vi "carrier_waveforms.vi"(5 "Modulation info":T8={"Fs full"=0.0, "Fs high"=0.0, "Fs low"=0.0, "Read size"=0, "FFT size low"=5000, "df low"=5000.0, "High carriers"=[], "Low carriers"=[], "Hi channels at low"=[7]} {"Hi channels at low" min=0 step=1; "Low carriers" format="%#_6p"; "High carriers" format="%#_6p"}, 6 "Freq response":bool, 7 "ilemt_config":T2={"IO params"={"Conversion"={"Rate"=4.0, "Num cards"=2, "Out channels"=4}, "Carriers"={"Phase shift"=180.0, "Levels"=[[0.8, 0.8, 0.8], [0.03, 0.03, 0.03]], "Delay samples"=73.15}, "TCP"={"Host"="192.168.1.15", "Port"=6666, "Buffering"=6, "Timeout"=6}, "Input channel sign"=[1, 1, 1]}, "High rate STFT"={"Win param"=101.5, "Window type"=61, "Win order"=2, "DFT size"=64, "Channels"=[7], "Oversample"=64}, "Low rate STFT"={"Win param"=120.0, "Window type"=61, "Win order"=8, "DFT size"=64, "Channels"=[7], "Oversample"=64}, "Filtering "=[]} {"Filtering"."Distortion"."Limit" format="%#_3p"; "Filtering"."Distortion"."LF cut" format="%#_3p"; "Filtering"."Kalman"."Measure noise" format="%#_3p"; "Filtering"."Kalman"."Process noise" format="%#_3p"; "Filtering"."Hum"."Limit" format="%#_3p"; "Filtering"."Hum"."Frequency" format="%#_4p"; "Low rate STFT"."Oversample" min=1 step=1; "Low rate STFT"."Channels" min=0 step=1; "Low rate STFT"."DFT size" min=1 step=1; "Low rate STFT"."Window type" items=["Rectangle"=0, "Hanning"=1, "Hamming"=2, "Blackman-Harris"=3, "Exact Blackman"=4, "Blackman"=5, "Flat Top"=6, "4 Term B-Harris "=7, "7 Term B-Harris"=8, "Low Sidelobe"=9, "Blackman Nuttall"=11, "Triangle"=30, "Bartlett-Hanning"=31, "Bohman"=32, "Parzen"=33, "Welch"=34, "Kaiser"=60, "Dolph-Chebyshev"=61, "Gaussian"=62]; "High rate STFT"."Oversample" min=1 step=1; "High rate STFT"."Channels" min=0 step=1; "High rate STFT"."DFT size" min=1 step=1; "High rate STFT"."Window type" items=["Rectangle"=0, "Hanning"=1, "Hamming"=2, "Blackman-Harris"=3, "Exact Blackman"=4, "Blackman"=5, "Flat Top"=6, "4 Term B-Harris "=7, "7 Term B-Harris"=8, "Low Sidelobe"=9, "Blackman Nuttall"=11, "Triangle"=30, "Bartlett-Hanning"=31, "Bohman"=32, "Parzen"=33, "Welch"=34, "Kaiser"=60, "Dolph-Chebyshev"=61, "Gaussian"=62]; "IO params"."Input channel sign" min=-1 max=1 step=1; "IO params"."Carriers"."Levels" min=0.0 step=0.1; "IO params"."Conversion"."Rate" format="%#_8g"}) -> (1 "Comp fault":bool, 2 "Output data":i32[][](array[numeric]), 3 "Source waveforms":waveform(dbl)[](graph))   [LabVIEW 2024]
uses:
  modulation_info.ctl
  ilemt_config.ctl
  system/IO_params.ctl
  stft_params.ctl
  <vilib>/Analysis/4window.llb/windowTd.ctl
  filter_params.ctl
  detrend_mode.ctl
  card_carrier_amplitudes.ctl
  <vilib>/Analysis/2dsp.llb/Inverse Real FFT.vi
  main/ilemt_globals.vi
  <vilib>/measure/NI_MABase.lvlib
  <vilib>/Analysis/NI_AALPro.lvlib
panel:
  in  "Comp fault threshold":dbl=0.2
  in  "Comp gain":dbl=0.05
  in  "Comp once":bool
  out "Compensated output":T1=[[[0.8395770614877774+0.0028758063900550953i, -0.018324423372348016-0.0006201934581264143i, -0.016886925649108726-2.940545835293518e-05i], [-0.01697562432214083-0.0016348024111330225i, 0.83885135156083+0.0020670504279334634i, -0.017173180533270275+0.00019269400281305392i], [-0.016374422884271427-0.0030083353945267676i, -0.0193629198646361-0.0014643391916366435i, 0.8367125904896281-0.0010501471602728106i]], [[0.03133897239102365+0.0006252328873188348i, -0.00048275091331450914-0.0003089130018055452i, -0.00043021631765542174-0.0002759884878732777i], [-0.0005913630072077795-0.00031200916130722737i, 0.03127992971510062+0.0004833529231568414i, -0.000494785304455945-0.0002579575827334465i], [-0.0007333860538198184-0.0003567516731933187i, -0.0006880917601750341-0.00033092556285938983i, 0.031083261126587918+0.00032228091837395326i]]] format="%#_3p"
  in  "Coupling comp":bool=TRUE
  # "Frequency response calibration mode"
  # "Parameters:"
  # "Gain used by auto-compensation of carrier cross coupling, <= 1. This is an integral gain."
  # "What fraction of the total carrier amplitude that the compensated carrier amplitude may differ from the uncompensated carrier amplitudes."
  # "Compensation on?"
  # "Trigger a compensation now, at gain 1."
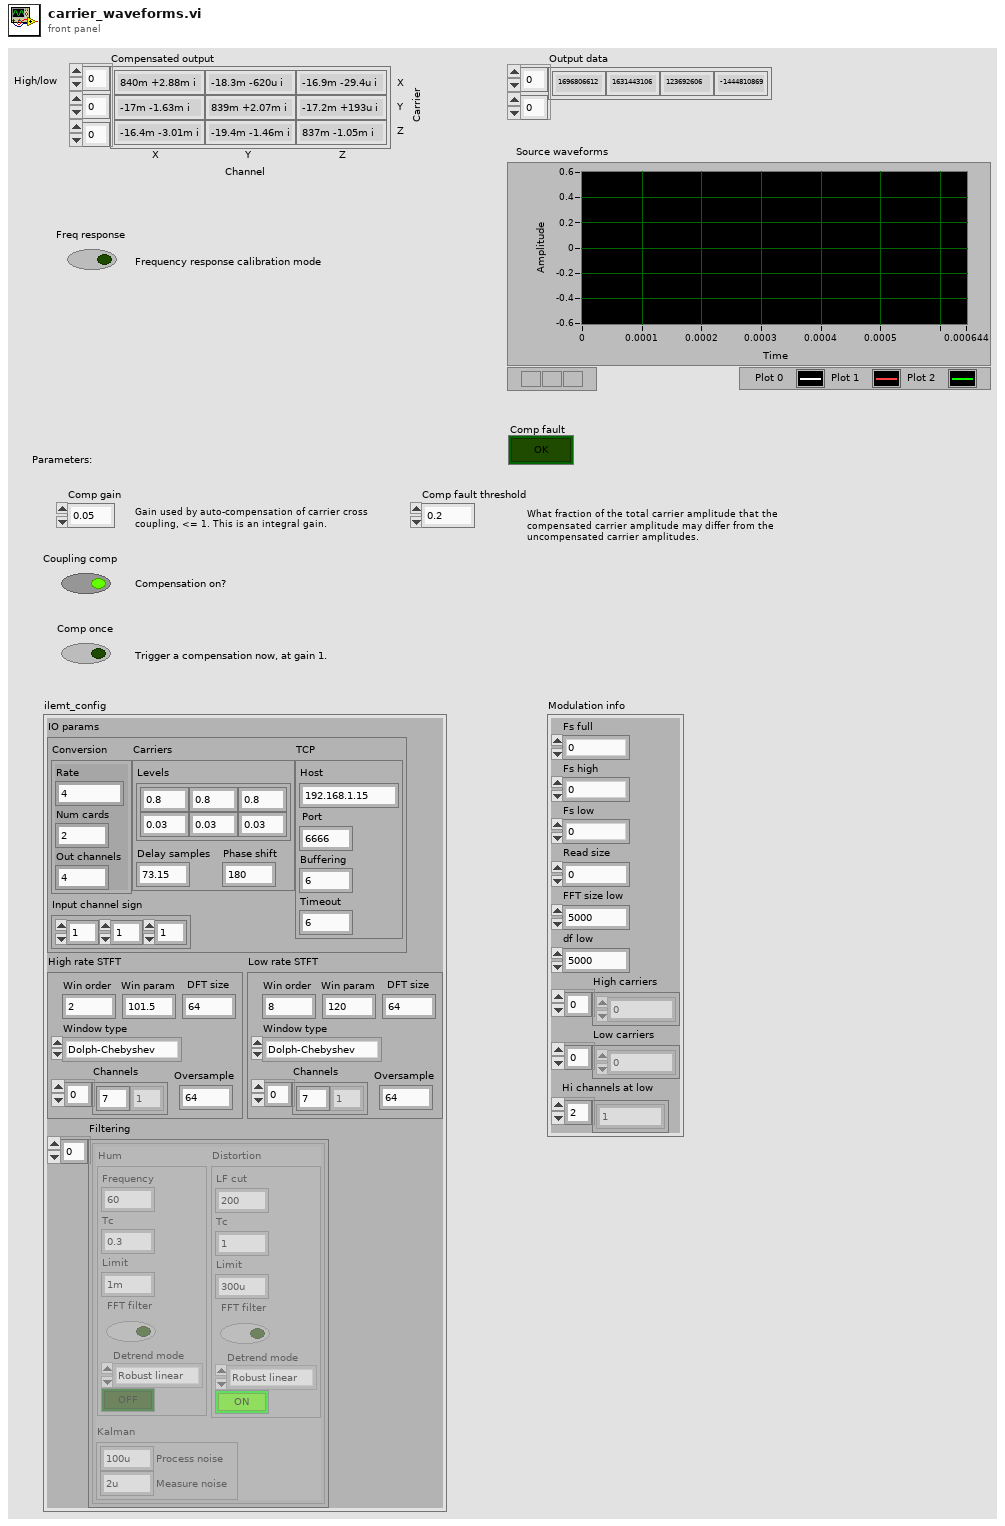
[diagram p1: front panel]
types:
  T1 = typedef "card_carrier_amplitudes.ctl" = cdb[][][]
  T2 = typedef "ilemt_config.ctl" = cluster{"IO params":T3, "High rate STFT":T4, "Low rate STFT":T4, "Filtering ":T6[]}
  T3 = typedef "IO_params.ctl" = cluster{"Conversion":cluster{"Rate":dbl, "Num cards":u32, "Out channels":u32}, "Carriers":cluster{"Phase shift":dbl, "Levels":dbl[][], "Delay samples":dbl}, "TCP":cluster{"Host":string, "Port":i32, "Buffering":u32, "Timeout":u32}, "Input channel sign":i32[]}
  T4 = typedef "stft_params.ctl" = cluster{"Win param":dbl, "Window type":T5, "Win order":i32, "DFT size":i32, "Channels":i32[], "Oversample":i32}
  T5 = typedef "NI_AALPro.lvlib/windowTd.ctl" = u32
  T6 = typedef "filter_params.ctl" = cluster{"Hum":cluster{"Frequency":dbl, "Tc":dbl, "Limit":dbl, "FFT filter":bool, "Detrend mode":T7, "Enable":bool}, "Kalman":cluster{"Process noise":dbl, "Measure noise":dbl}, "Distortion":cluster{"LF cut":dbl, "Tc":dbl, "Limit":dbl, "FFT filter":bool, "Detrend mode":T7, "Enable":bool}}
  T7 = typedef "detrend_mode.ctl" = enum16{"Zero mean", "Linear", "Robust linear"}
  T8 = typedef "modulation_info.ctl" = cluster{"Fs full":dbl, "Fs high":dbl, "Fs low":dbl, "Read size":i32, "FFT size low":i32, "df low":dbl, "High carriers":dbl[], "Low carriers":dbl[], "Hi channels at low":i32[]}
  T9 = typedef "carrier_amplitudes.ctl" = cdb[][][][]
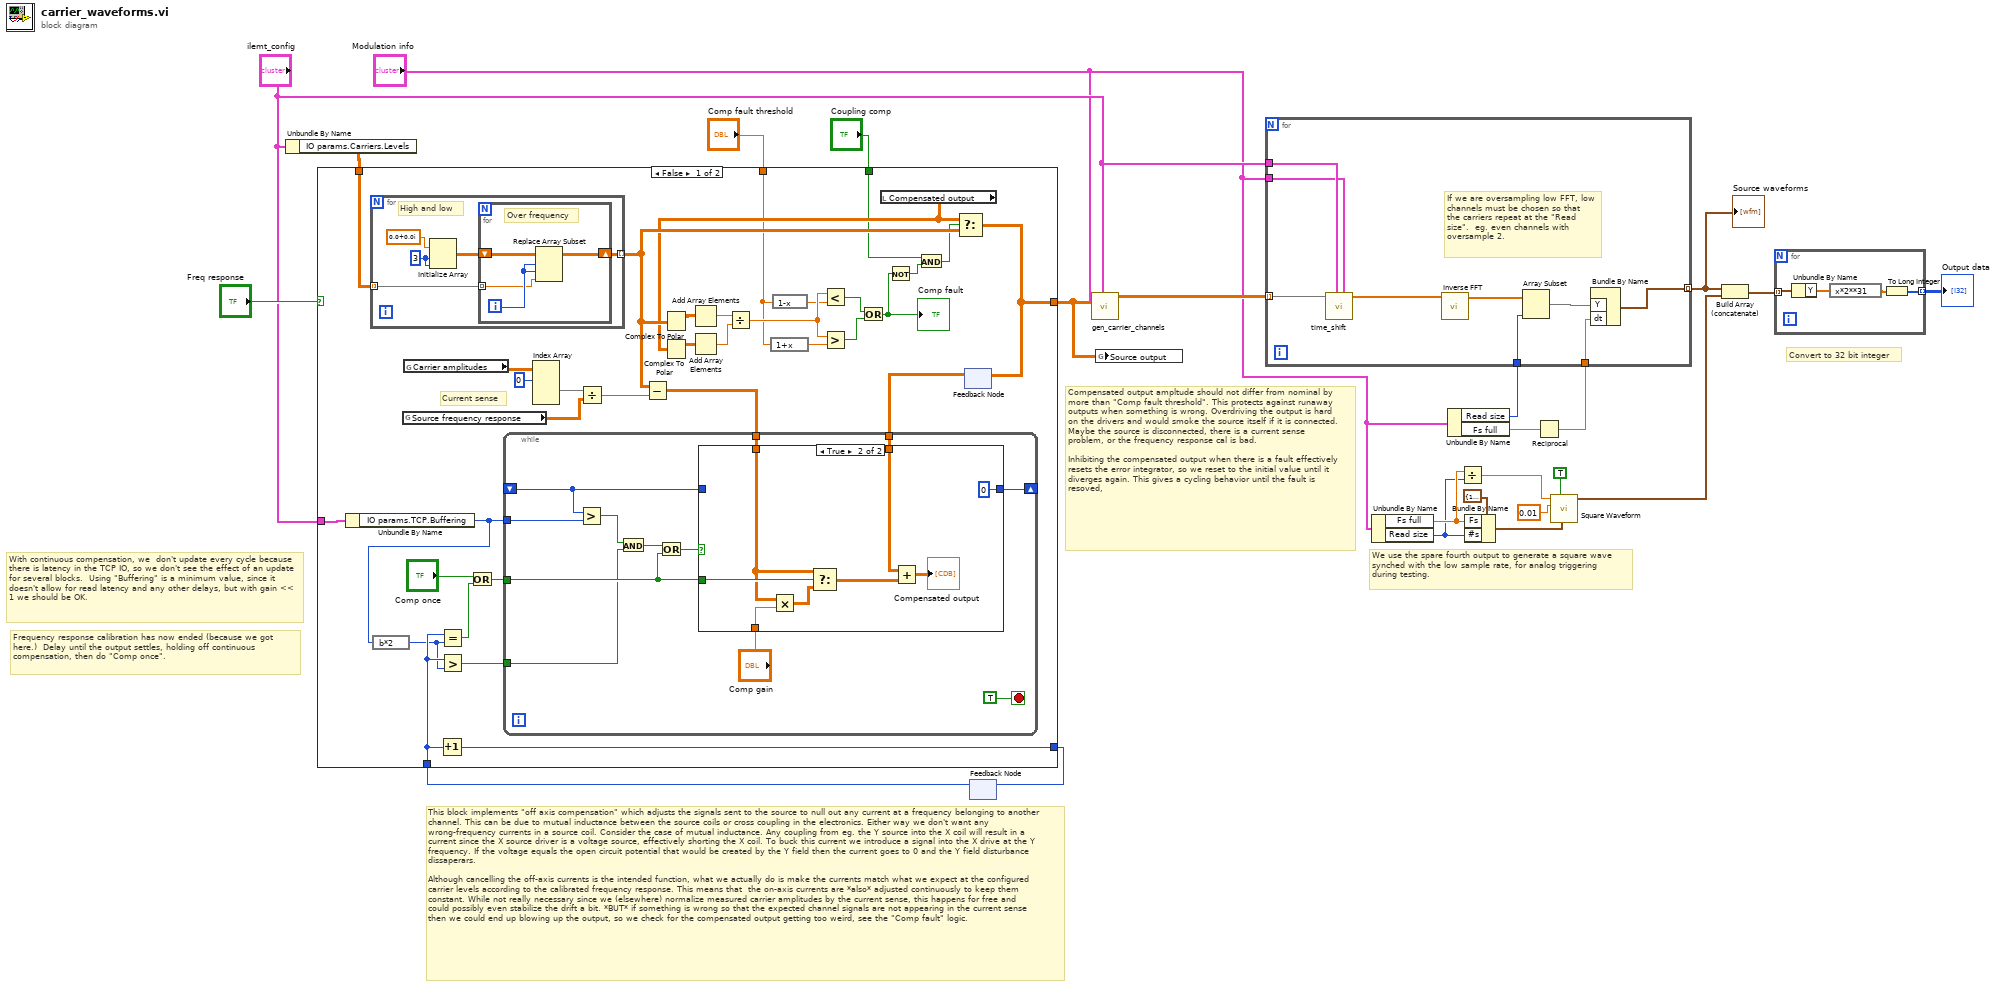
[diagram p0: block diagram]
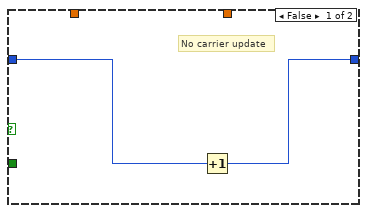
[diagram p2: hidden frame]
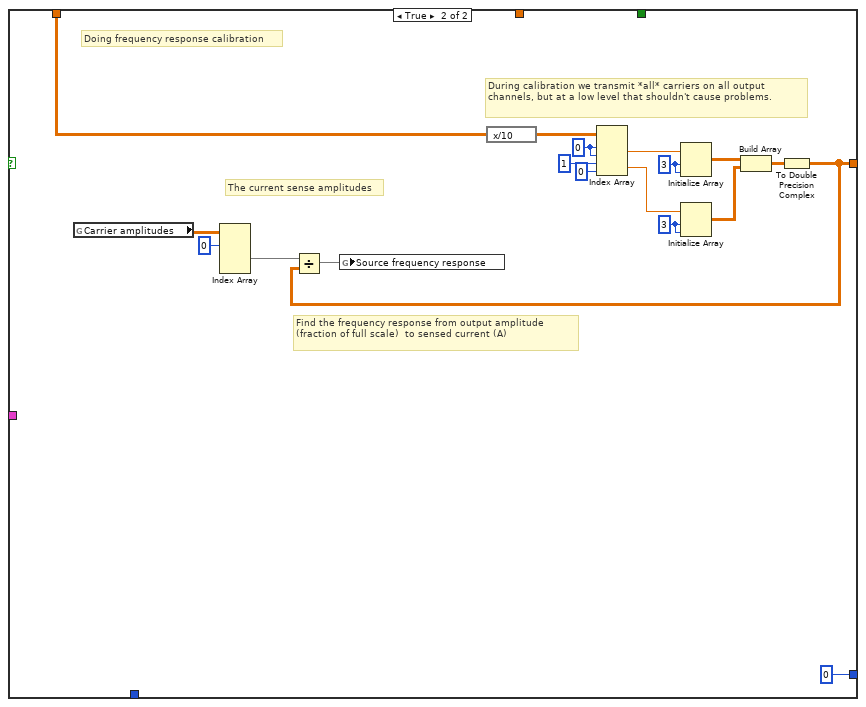
[diagram p3: hidden frame]
diagram:
  # "This block implements \"off axis compensation\" which adjusts the signals sent to the source to null out any current at a frequency belonging to another channel. This can be due to mutual inductance between the source coils or cross coupling in the electronics. Either way we don't want any wrong-frequency currents in a source coil. Consider the case of mutual inductance. Any coupling from eg. the Y source into the X coil will result in a current since the X source driver is a voltage source, effectively shorting the X coil. To buck this current we introduce a signal into the X drive at the Y frequency. If the voltage equals the open circuit potential that would be created by the Y field then the current goes to 0 and the Y field disturbance dissaperars.\n\nAlthough cancelling the off-axis currents is the intended function, what we actually do is make the currents match what we expect at the configured carrier levels according to the calibrated frequency response. This means that  the on-axis currents are *also* adjusted continuously to keep them constant. While not really necessary since we (elsewhere) normalize measured carrier amplitudes by the current sense, this happens for free and could possibly even stabilize the drift a bit. *BUT* if something is wrong so that the expected channel signals are not appearing in the current sense then we could end up blowing up the output, so we check for the compensated output getting too weird, see the \"Comp fault\" logic."
  # "Compensated output ampltude should not differ from nominal by more than \"Comp fault threshold\". This protects against runaway outputs when something is wrong. Overdriving the output is hard on the drivers and would smoke the source itself if it is connected. Maybe the source is disconnected, there is a current sense problem, or the frequency response cal is bad.\n\nInhibiting the compensated output when there is a fault effectively resets the error integrator, so we reset to the initial value until it diverges again. This gives a cycling behavior until the fault is resoved,"
  # "Frequency response calibration has now ended (because we got here.)  Delay until the output settles, holding off continuous compensation, then do \"Comp once\"."
  # "With continuous compensation, we  don't update every cycle because there is latency in the TCP IO, so we don't see the effect of an update for several blocks.  Using \"Buffering\" is a minimum value, since it doesn't allow for read latency and any other delays, but with gain << 1 we should be OK."
  # "Convert to 32 bit integer"
  # "We use the spare fourth output to generate a square wave synched with the low sample rate, for analog triggering during testing."
  n1 = Unbundle By Name("ilemt_config") -> ("IO params.Carriers.Levels"=w9:dbl[][])
  n2 = feedback #1() -> (w4:i32)  [unwired: 1 in]
  n3 = case shown="False" "Freq response" {
    tunnel: w9 -> [w58 w92]
    tunnel: [w53 w90] -> w7
    tunnel: "ilemt_config" -> [w52 _]
    tunnel: [w50 0 ("Read size")] -> w5
    tunnel: w4 -> [w45 _]
    tunnel: "Coupling comp" -> [w28 _]
    tunnel: "Comp fault threshold" -> [w25 _]
    frame False {
      # "Current sense"
      n4 = Unbundle By Name(w52) -> ("IO params.TCP.Buffering"=w49:u32)
      n5 = for {
        tunnel: w58 -> [w82] mode=indexing
        tunnel: [w81] -> w40 mode=indexing
        w85 = 3 ("dimension size")
        # "High and low"
        n6 = Initialize Array(cdb 0.0+0.0i, w85, w85) -> (w83:cdb[][])
        n7 = for {
          tunnel: w82 -> [w87] mode=indexing
          shift-right: [w86] -> w81
          shift-left: w83 -> [w89]
          i -> [w88]
          # "Over frequency"
          n8 = Replace Array Subset(array=w89, new element=w87, index (row)=w88, index (col)=w88) -> (w86:cdb[][])
        }
      }
      n9 = expression code="b*2"(w49) -> (w44:u32)
      n10 = global read "ilemt_globals.vi" "Source frequency response"() -> (w54:T1)
      n11 = global read "ilemt_globals.vi" "Carrier amplitudes"() -> (w57:T9)
      n12 = Increment(x=w45) -> (x+1=w50:i32)
      n13 = Equal?(x=w45, y=w44) -> (x = y?=w47:bool)
      n14 = Greater?(x=w45, y=w44) -> (0:w43:bool)
      n15 = Or(x="Comp once", y=w47) -> (x .or. y?=w46:bool)
      n16 = Index Array(array=w57, index (dim 0)=0 ("index (vol)")) -> (element=w55:cdb[][][])  [unwired: 3 in]
      n17 = Divide(x=w55, y=w54) -> (x/y=w37:cdb[][][])
      n18 = Subtract(x=w40, y=w37) -> (x-y=w51:cdb[][][])
      n19 = Complex To Polar(r * e^(i*theta)=w40) -> (r=w39:dbl[][][])  [unwired: 1 out]
      n20 = Add Array Elements(numeric array=w39) -> (sum=w42:dbl)
      n21 = expression code="1+x"(w25) -> (w27:dbl)
      n22 = expression code="1-x"(w25) -> (w26:dbl)
      n23 = local read "Compensated output"() -> (w29:T1)
      n24 = Complex To Polar(r * e^(i*theta)=w29) -> (r=w38:dbl[][][])  [unwired: 1 out]
      n25 = Add Array Elements(numeric array=w38) -> (sum=w41:dbl)
      n26 = Divide(x=w42, y=w41) -> (x/y=w36:dbl)
      n27 = Less?(x=w36, y=w26) -> (x < y?=w34:bool)
      n28 = Greater?(x=w36, y=w27) -> (0:w35:bool)
      n29 = Or(x=w34, y=w35) -> (x .or. y?=w33:bool)
      "Comp fault" <- w33
      n30 = Not(x=w33) -> (.not. x?=w32:bool)
      n31 = And(x=w28, y=w32) -> (x .and. y?=w31:bool)
      n32 = Select(t=w29, s=w31, f=w40) -> (s? t:f=w53:T1)
      n33 = feedback-in #2(w53) -> ()
      n34 = feedback #2() -> (w30:T1)  [unwired: 1 in]
      n35 = while {
        tunnel: w46 -> [w65]
        shift-right: [w67] -> _
        shift-left: _ -> [w68]
        tunnel: w49 -> [w69]
        tunnel: w30 -> [w66]
        tunnel: w51 -> [w64]
        tunnel: w43 -> [w60]
        stop <- TRUE stop-if-true
        n36 = Greater?(x=w68, y=w69) -> (0:w62:bool)
        n37 = And(x=w62, y=w60) -> (x .and. y?=w61:bool)
        n38 = Or(x=w61, y=w65) -> (x .or. y?=w59:bool)
        n39 = case shown="True" w59 {
          tunnel: w68 -> [w72 _]
          tunnel: [w71 0] -> w67
          tunnel: w66 -> [_ w79]
          tunnel: w65 -> [_ w77]
          tunnel: w64 -> [_ w75]
          tunnel: "Comp gain" -> [_ w73]
          frame False {
            # "No carrier update"
            n40 = Increment(x=w72) -> (x+1=w71:i32)
          }
          frame True {
            n41 = Multiply(x=w75, y=w73) -> (x*y=w74:cdb[][][])
            n42 = Select(t=w75, s=w77, f=w74) -> (s? t:f=w76:cdb[][][])
            n43 = Add(x=w79, y=w76) -> (x+y=→"Compensated output":T1)
          }
        }
      }
    }
    frame True {
      w98 = 0 ("index (row)")
      w106 = 3 ("dimension size")
      w107 = 3 ("dimension size")
      # "Find the frequency response from output amplitude (fraction of full scale)  to sensed current (A)"
      # "The current sense amplitudes"
      # "During calibration we transmit *all* carriers on all output channels, but at a low level that shouldn't cause problems."
      # "Doing frequency response calibration"
      n44 = global read "ilemt_globals.vi" "Carrier amplitudes"() -> (w103:T9)
      n45 = Index Array(array=w103, index (dim 0)=0 ("index (vol)")) -> (element=w101:cdb[][][])  [unwired: 3 in]
      n46 = expression code="x/10"(w92) -> (w93:dbl[][])
      n47 = Index Array(array=w93, index (row) #1=w98, index (col) #1=w98, index (row) #2=1 ("index (row)"), index (col) #2=0 ("disabled index (col)")) -> (element #1=w95:dbl, element #2=w94:dbl)
      n48 = Initialize Array(w95, w107, w107) -> (w105:dbl[][])
      n49 = Initialize Array(w94, w106, w106) -> (w104:dbl[][])
      n50 = Build Array(w105, w104) -> (w91:dbl[][][])
      n51 = To Double Precision Complex(1:w91) -> (0:w90:cdb[][][])
      n52 = Divide(x=w101, y=w90) -> (x/y=w100:cdb[][][])
      n53 = global write "ilemt_globals.vi" "Source frequency response"(w100) -> ()
    }
  }
  n54 = feedback-in #1(w5) -> ()
  n55 = call "gen_carrier_channels.vi"("Modulation info"="Modulation info", "ilemt_config"="ilemt_config", "Source amplitudes"=w7) -> ("Carrier DFT"=w10:cdb[][])  [unwired: 8 in]
  n56 = global write "ilemt_globals.vi" "Source output"(w7) -> ()
  n57 = Unbundle By Name("Modulation info") -> ("Fs full"=w23:dbl, "Read size"=w11:i32)
  n58 = Unbundle By Name("Modulation info") -> ("Read size"=w14:i32, "Fs full"=w13:dbl)
  n59 = Divide(x=w23, y=w11) -> (x/y=w20:dbl)
  n60 = Bundle By Name(cluster=cluster{"Fs":dbl, "#s":dbl} {"Fs"=1000.0, "#s"=1000.0} ("sampling info"), "Fs"=w23, "#s"=w11) -> (w21:cluster{"Fs":dbl, "#s":dbl})
  n61 = Reciprocal(x=w13) -> (1/x=w12:dbl)
  n62 = for {
    tunnel: [w116] -> w17 mode=indexing
    tunnel: w14 -> [w112]
    tunnel: w12 -> [w111]
    tunnel: "ilemt_config" -> [w110]
    tunnel: "Modulation info" -> [w109]
    tunnel: w10 -> [w108] mode=indexing
    # "If we are oversampling low FFT, low channels must be chosen so that the carriers repeat at the \"Read size\".  eg. even channels with oversample 2."
    n63 = call "time_shift.vi"("Modulation info"=w109, "ilemt_config"=w110, "Array in"=w108) -> ("Array out"=w113:cdb[])  [unwired: 8 in]
    n64 = call-poly <vilib>:"Inverse FFT.vi"("FFT {X}"=w113) -> ("X"=w115:dbl[])  [unwired: 9 in, 1 out]
    n65 = Array Subset(array=w115, length=w112) -> (w114:dbl[])  [unwired: 1 in]
    n66 = Bundle By Name("Y"=w114, "dt"=w111) -> (w116:waveform(dbl))  [unwired: 1 in]
  }
  "Source waveforms" <- w17
  n67 = call <vilib>:"Square Waveform.vi"("sampling info"=w21, "reset signal"=TRUE, "amplitude"=0.01, "frequency"=w20) -> ("signal out"=w18:waveform(dbl))  [unwired: 6 in, 1 out]
  n68 = Build Array (concatenate)(w17, w18) -> (w16:waveform(dbl)[])
  n69 = for {
    tunnel: w16 -> [w120] mode=indexing
    tunnel: [w117] -> w15 mode=indexing
    n70 = Unbundle By Name(w120) -> ("Y"=w119:dbl[])
    n71 = expression code="x*2**31"(w119) -> (w118:dbl[])
    n72 = To Long Integer(number=w118) -> (32bit integer=w117:i32[])
  }
  "Output data" <- w15
